vi "main_ctrl.vi"(8 "error in":errorcluster) -> (0 "error out":errorcluster caption="Error")   [LabVIEW 2013]
uses:
  <vilib>/Rock Robotics/WPI/DriverStation/WPI_DriverStationRobotMode2.ctl
  typedefs/fg_typedef.ctl
  typedefs/vision enable.ctl
  typedefs/vision data.ctl
  typedefs/subStates.ctl
  typedefs/singleUseSubstate.ctl
  <vilib>/Rock Robotics/WPI/Solenoid/WPI_SolenoidValue.ctl
  <vilib>/Rock Robotics/WPI/Compressor/WPI_CompressorGetSetRefNum.vi
  <vilib>/Rock Robotics/WPI/RobotDrive/WPI_RobotDriveGetSetRefNum.vi
  <vilib>/Rock Robotics/WPI/RobotDrive/WPI_RobotDriveArcadeDrive_Standard(NoSaturation).vi
  <vilib>/Rock Robotics/WPI/Solenoid/WPI_SolenoidSetEnum.vi
panel:
  out "Robot Mode":T1
  out "Vision SPI":u32
  out "Vision IPS":dbl
  out "Main IPS":dbl
  out "Main SPI":u32
  # "MAIN CONTROL"
  # "holds robot control code - dual parallel state machine"
  # "SPI: milliseconds per iteration\nIPS: iterations per second"
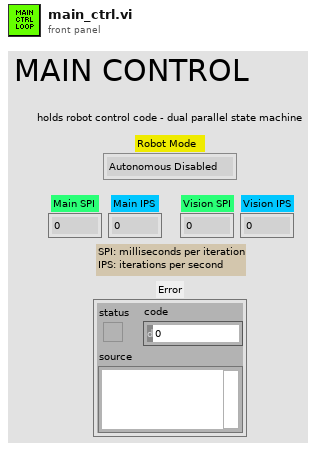
[diagram p1: front panel]
types:
  T1 = typedef "WPI_DriverStationRobotMode2.ctl" = enum16{"Autonomous Disabled", "Autonomous Enabled", "Teleop Disabled", "Teleop Enabled", "Timeout", "Finish", "Test Disabled", "Test Enabled"}
  T2 = typedef "fg_typedef.ctl" = enum16{"Get", "Set"}
  T3 = typedef "WPI_RobotDriveDevRef.ctl" = cluster{"DevStatus":errorcluster, "Motors[]":T4[], "Square Inputs":bool, "Max Output":dbl, "Isochronous":bool}
  T4 = typedef "WPI_MotorControlDeviceRef.ctl" = cluster{"DeviceStatus":errorcluster, "Type":enum16{"PWM", "CAN"}, "PWM":cluster{"Digital Module":T5, "PWM Channel":T6, "DeadBand":T7}, "CAN":cluster{"Device Number":u8, "Control Mode":T8, "Semaphore":T9, "Max Vout":dbl}, "Invert":bool, "TransformRef":T10, "InvTransformRef":T10}
  T5 = typedef "FPGA_TypedefDigitalModule.ctl" = enum16{"Digital Module 1", "Digital Module 2"}
  T6 = typedef "FPGA_DIOPWMChannel.ctl" = enum8{"PWM 1", "PWM 2", "PWM 3", "PWM 4", "PWM 5", "PWM 6", "PWM 7", "PWM 8", "PWM 9", "PWM 10", "Invalid"}
  T7 = typedef "WPI_PWMDeadband.ctl" = cluster{"Name":string, "maxPositivePwm":i32, "minPositivePwm":i32, "centerPwm":i32, "maxNegativePwm":i32, "minNegativePwm":i32, "angularRange":u16}
  T8 = typedef "WPI_CANJaguar_ControlMode.ctl" = enum8{"Percent VBus", "Current", "Speed", "Position", "Voltage"}
  T9 = typedef "Semaphore RefNum" = refnum<k1>
  T10 = typedef "WPI_PWMTransform_ConPane.ctl" = refnum<vi>
  T11 = typedef "WPI_SolenoidDevRef.ctl" = cluster{"DevStatus":errorcluster, "Solenoid Module":T12, "Forward Solenoid Channel":T13, "Reverse Solenoid Channel":T13}
  T12 = typedef "FPGA_TypedefSolenoidModule.ctl" = enum16{"Solenoid Module 1", "Solenoid Module 2"}
  T13 = typedef "WPI_SolenoidChannel.ctl" = enum8{"Solenoid 1", "Solenoid 2", "Solenoid 3", "Solenoid 4", "Solenoid 5", "Solenoid 6", "Solenoid 7", "Solenoid 8", "Invalid"}
  T14 = typedef "WPI_DigitalInputDevRef.ctl" = cluster{"DevStatus":errorcluster, "DIO Channel":T15, "Digital Module":T5}
  T15 = typedef "FPGA_DIOChannel.ctl" = enum8{"DIO 1", "DIO 2", "DIO 3", "DIO 4", "DIO 5", "DIO 6", "DIO 7", "DIO 8", "DIO 9", "DIO 10", "DIO 11", "DIO 12", "DIO 13", "DIO 14", "Invalid"}
  T16 = typedef "WPI_EncoderDevRef.ctl" = cluster{"DevStatus":errorcluster, "EncoderIndex":T17, "CounterIndex":T18, "DistancePerCount":dbl, "Decoding Type":T19}
  T17 = typedef "FPGA_EncoderIdx.ctl" = enum8{"Enc 0", "Enc 1", "Enc 2", "Enc 3", "Invalid"}
  T18 = typedef "FPGA_CounterCtrSystemIndex.ctl" = enum8{"Ctr 0", "Ctr 1", "Ctr 2", "Ctr 3", "Ctr 4", "Ctr 5", "Ctr 6", "Ctr 7", "Invalid"}
  T19 = typedef "WPI_EncoderType.ctl" = enum16{"1x", "2x", "4x"}
  T20 = typedef "vision data.ctl" = cluster{"x":dbl, "y":dbl, "area":dbl, "width":dbl, "height":dbl, "Hot Goal Present?":bool, "distance":dbl}
  T21 = typedef "vision enable.ctl" = enum16{"Enable", "Disable", "Stop"}
  T22 = typedef "WPI_CameraDevRef.ctl" = cluster{"Camera Address":string, "CameraStatus":errorcluster, "Acquire Image Notifier":refnum<notifier>}
  T23 = typedef "IMAQ Image.ctl" = refnum<image>
  T24 = cluster{"Vision mSPI":u32, "Main mSPI":u32, "Dash mSPI":u32}
  T25 = typedef "WPI_CompressorDevRef.ctl" = cluster{"DevStatus":errorcluster, "DigitalInputDevRef":T14, "RelayDevRef":T26}
  T26 = typedef "WPI_RelayDevRef.ctl" = cluster{"DevStatus":errorcluster, "Relay Channel":T27, "Digital Module":T5, "Relay Direction":T28}
  T27 = typedef "FPGA_DIORelayChannel.ctl" = enum8{"Relay 1", "Relay 2", "Relay 3", "Relay 4", "Relay 5", "Relay 6", "Relay 7", "Relay 8", "Invalid"}
  T28 = typedef "WPI_RelayDirection.ctl" = enum16{"Both directions", "Forward only", "Reverse only"}
  T29 = typedef "WPI_SolenoidValue.ctl" = enum16{"Off", "On", "Forward", "Reverse"}
  T30 = typedef "singleUseSubstate.ctl" = enum16{"null", "wait", "shift high", "shift low", "extend shooter", "retract shooter", "latch", "unlatch"}
  T31 = typedef "WPI_DriverStationDerivedRobotMode.ctl" = enum16{"Init", "Execute", "Stop"}
  T32 = typedef "subStates.ctl" = enum16{"null", "wait", "driver control", "auto", "manual override", "hold position", "rotate", "pickup", "pass", "load", "goto shoot", "shoot high goal", "shoot low goal", "cancel arm", "cancel shooter", "end"}
  T33 = typedef "Loop 2 Datatype.ctl" = cluster{"State":T32, "Waiting Loop":i32, "State to Wait For":i32, "Loop ID":i32, "Exit Value":i32, "Joystick Y":dbl, "Joystick Z":dbl}
  T34 = typedef "Loop 1 Datatype.ctl" = cluster{"State":T32, "Waiting Loop":i32, "State to Wait For":i32, "Loop ID":i32, "Exit Value":i32}
  T35 = typedef "Loop 3 Datatype.ctl" = cluster{"State":T32, "Waiting Loop":i32, "State to Wait For":i32, "Loop ID":i32, "Exit Value":i32, "Joystick Y":dbl, "Tune Setpoint":cluster{"Increment":bool, "Decrement":bool}}
  T36 = typedef "Loop 0 Datatype.ctl" = cluster{"State":T32, "Waiting Loop":i32, "State to Wait For":i32, "Loop ID":i32, "Exit Value":i32, "X Axis":dbl, "Y Axis":dbl, "Z Axis":dbl}
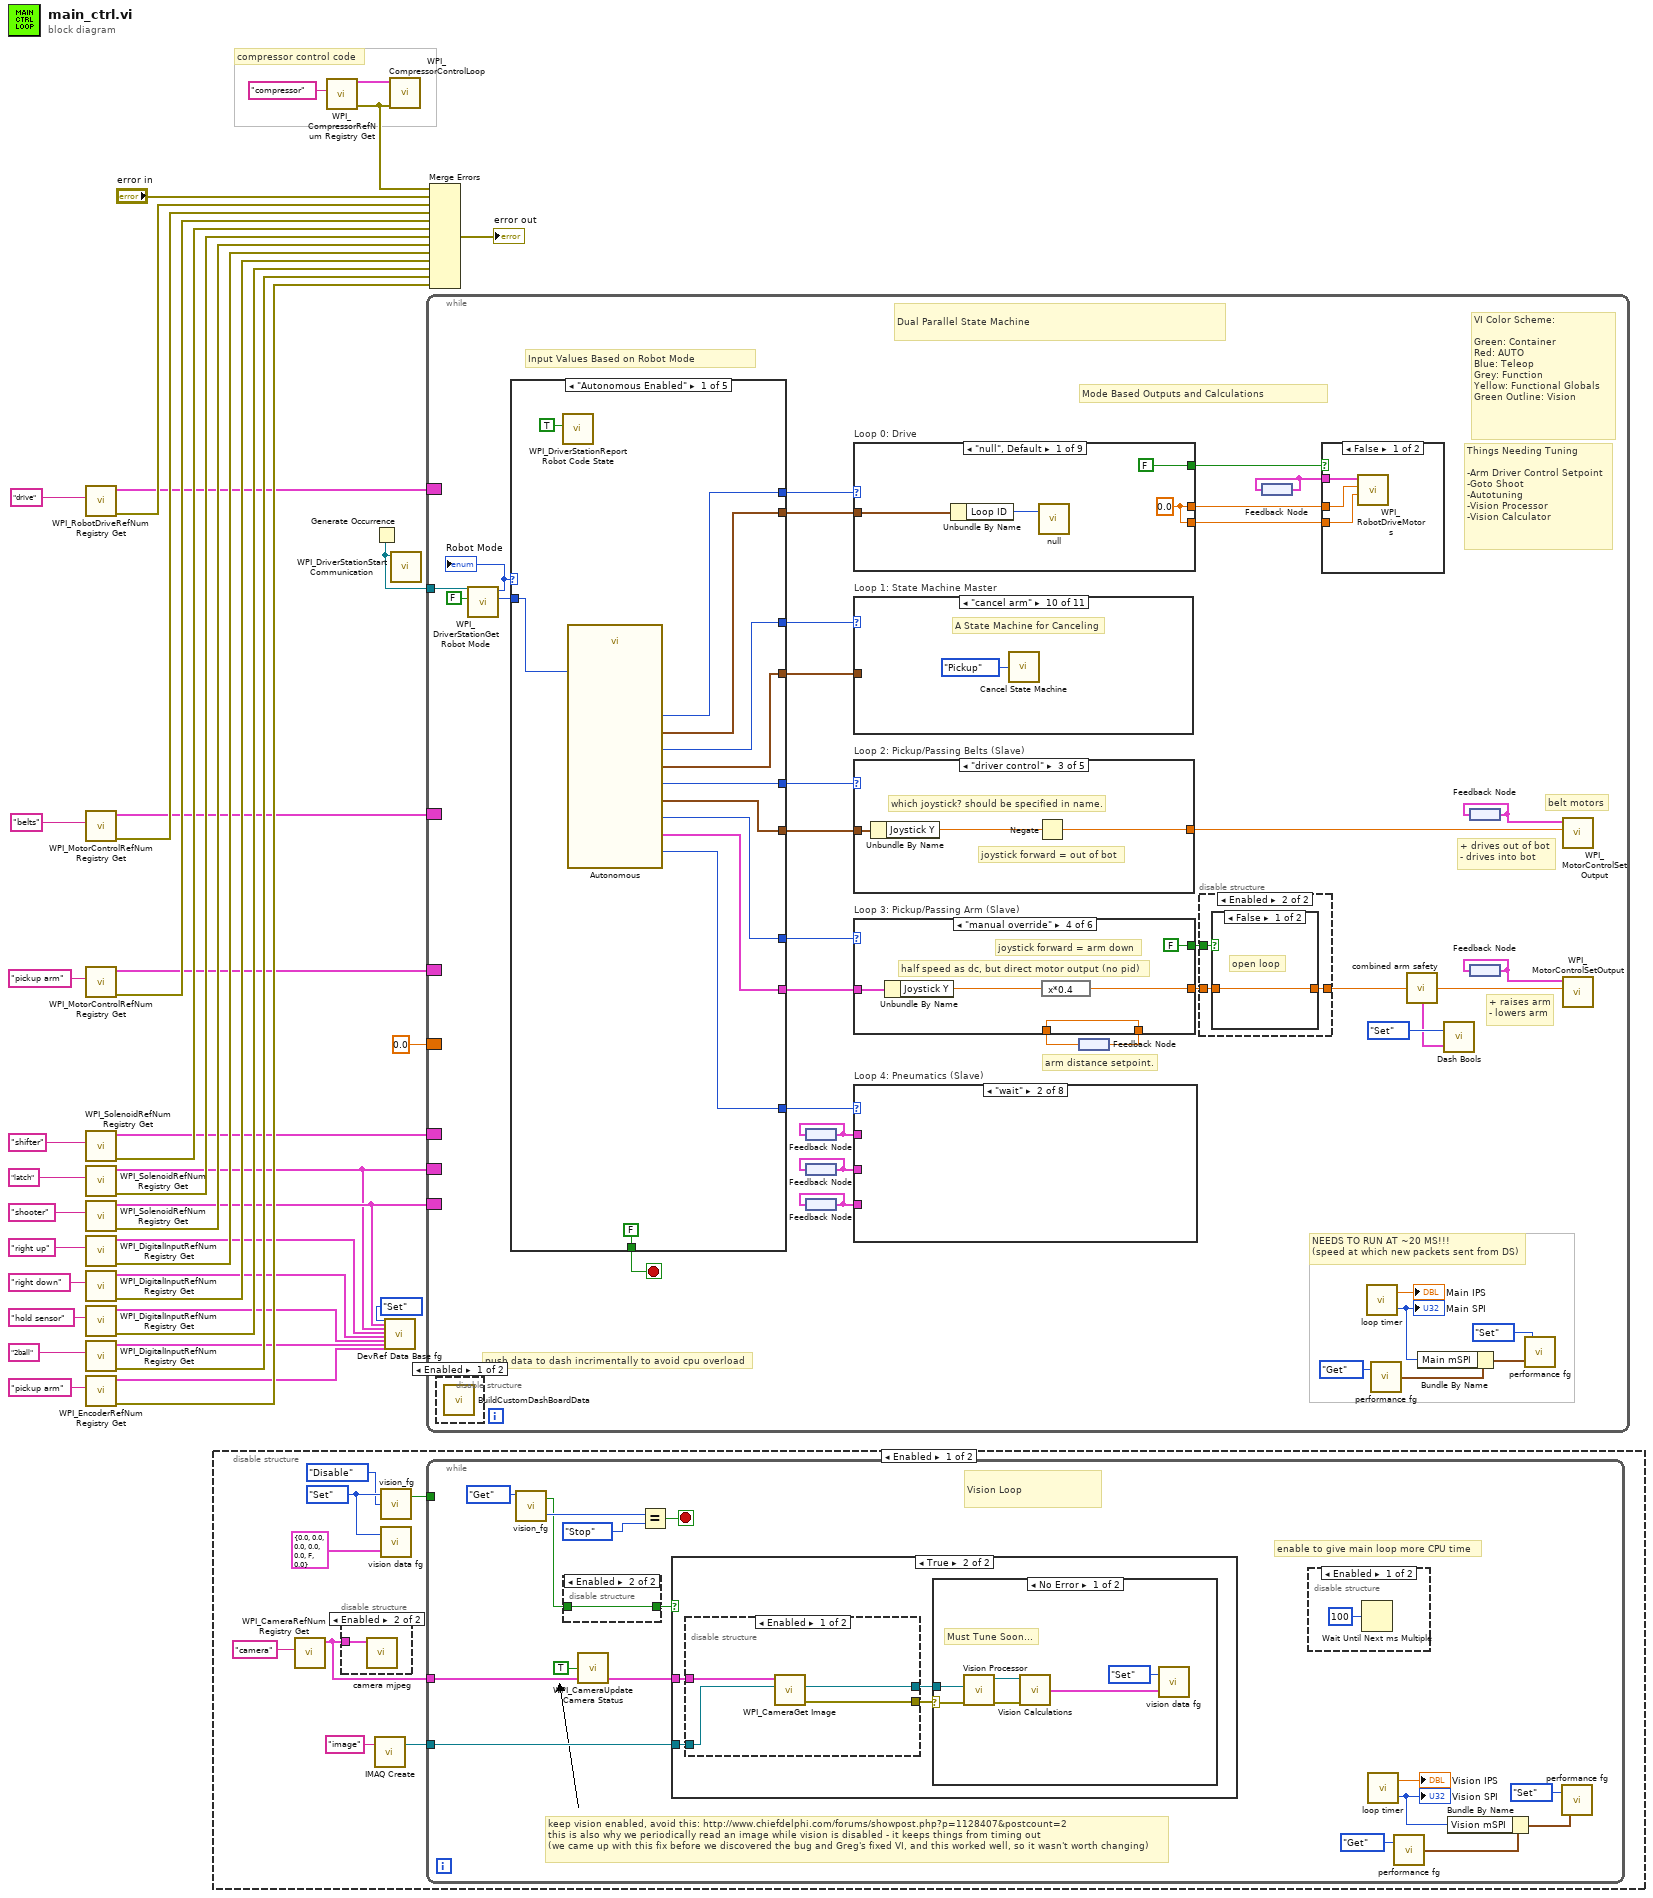
[diagram p0: block diagram]
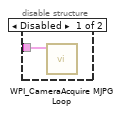
[diagram p2: hidden frame]
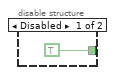
[diagram p3: hidden frame]
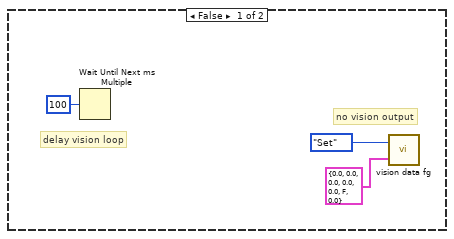
[diagram p5: hidden frame]
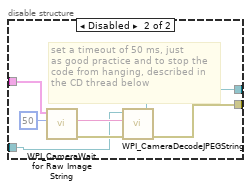
[diagram p7: hidden frame]
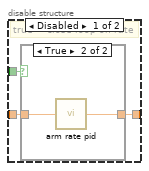
[diagram p9: hidden frame]
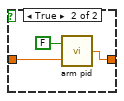
[diagram p11: hidden frame]
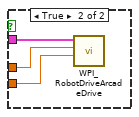
[diagram p13: hidden frame]
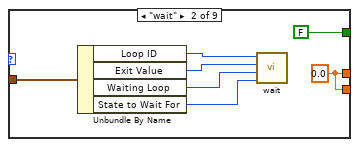
[diagram p14: hidden frame]
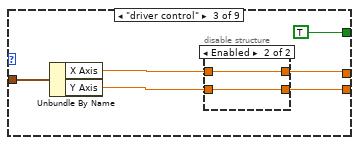
[diagram p15: hidden frame]
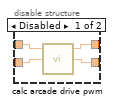
[diagram p16: hidden frame]
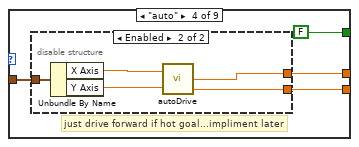
[diagram p17: hidden frame]
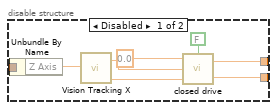
[diagram p18: hidden frame]
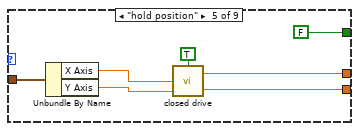
[diagram p19: hidden frame]
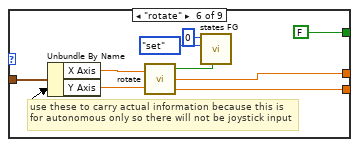
[diagram p20: hidden frame]
diagram:
  # "compressor control code"
  n1 = call <vilib>:"WPI_RobotDriveRefNum Registry Get.vi"("refnum name"="drive") -> ("error out"=w39:errorcluster, "RobotDriveDevRef"=w27:T3)  [unwired: 9 in]
  n2 = call <vilib>:"WPI_MotorControlRefNum Registry Get.vi"("refnum name"="belts") -> ("error out"=w38:errorcluster, "MotorControlDevRef"=w1:T4)  [unwired: 9 in]
  n3 = call <vilib>:"WPI_MotorControlRefNum Registry Get.vi"("refnum name"="pickup arm") -> ("error out"=w37:errorcluster, "MotorControlDevRef"=w18:T4)  [unwired: 9 in]
  n4 = call <vilib>:"WPI_SolenoidRefNum Registry Get.vi"("refnum name"="shifter") -> ("error out"=w36:errorcluster, "SolenoidDevRef"=w25:T11)  [unwired: 9 in]
  n5 = call <vilib>:"WPI_SolenoidRefNum Registry Get.vi"("refnum name"="latch") -> ("error out"=w35:errorcluster, "SolenoidDevRef"=w13:T11)  [unwired: 9 in]
  n6 = call <vilib>:"WPI_SolenoidRefNum Registry Get.vi"("refnum name"="shooter") -> ("error out"=w34:errorcluster, "SolenoidDevRef"=w14:T11)  [unwired: 9 in]
  n7 = call <vilib>:"WPI_DigitalInputRefNum Registry Get.vi"("refnum name"="right up") -> ("error out"=w33:errorcluster, "DigitalInputDevRef"=w12:T14)  [unwired: 9 in]
  n8 = call <vilib>:"WPI_DigitalInputRefNum Registry Get.vi"("refnum name"="right down") -> ("error out"=w32:errorcluster, "DigitalInputDevRef"=w11:T14)  [unwired: 9 in]
  n9 = call <vilib>:"WPI_DigitalInputRefNum Registry Get.vi"("refnum name"="hold sensor") -> ("error out"=w31:errorcluster, "DigitalInputDevRef"=w8:T14)  [unwired: 9 in]
  n10 = call <vilib>:"WPI_DigitalInputRefNum Registry Get.vi"("refnum name"="2ball") -> ("error out"=w40:errorcluster, "DigitalInputDevRef"=w3:T14)  [unwired: 9 in]
  n11 = call <vilib>:"WPI_EncoderRefNum Registry Get.vi"("refnum name"="pickup arm") -> ("error out"=w41:errorcluster, "EncoderDevRef"=w2:T16)  [unwired: 9 in]
  n12 = disable-structure shown="Enabled" {
    frame Enabled {
      w47 = fg_typedef."Set" ("Enum")
      n13 = call <vilib>:"WPI_CameraRefNum Registry Get.vi"("refnum name"="camera") -> ("CameraDevRef"=w44:T22)  [unwired: 9 in, 1 out]
      n14 = disable-structure shown="Enabled" {
        disable-tunnel: w44 -> [w50 w51]
        frame Disabled {
          n15 = call <vilib>:"WPI_CameraAcquire MJPG Loop.vi"("CameraDevRef"=w50) -> ()  [unwired: 11 in]
        }
        frame Enabled {
          n16 = call "camera mjpeg.vi"("CameraDevRef"=w51) -> ()  [unwired: 11 in]
        }
      }
      n17 = call "IMAQ Create"("Image Name"="image") -> ("New Image"=w49:T23)  [unwired: 4 in, 1 out]
      n18 = call "vision_fg.vi"("Action"=vision_enable."Disable", "Menu"=w47) -> ("Enabled?"=w48:bool)  [unwired: 1 in, 1 out]
      n19 = call "vision data fg.vi"("Input"=T20 {"x"=0.0, "y"=0.0, "area"=0.0, "width"=0.0, "height"=0.0, "Hot Goal Present?"=FALSE, "distance"=0.0} ("Cluster"), "Menu"=w47) -> ()  [unwired: 1 out]
      n20 = while {
        tunnel: w49 -> [w66]
        tunnel: w44 -> [w65]
        tunnel: w48 -> [_]
        stop <- w67 stop-if-true
        # "keep vision enabled, avoid this: http://www.chiefdelphi.com/forums/showpost.php?p=1128407&postcount=2\nthis is also why we periodically read an image while vision is disabled - it keeps things from timing out\n(we came up with this fix before we discovered the bug and Greg's fixed VI, and this worked well, so it wasn't worth changing)"
        # "enable to give main loop more CPU time"
        # "Vision Loop"
        n21 = call "vision_fg.vi"("Menu"=fg_typedef."Get" ("Enum")) -> ("State Out"=w61:T21, "Enabled?"=w52:bool)  [unwired: 2 in]
        n22 = disable-structure shown="Enabled" {
          disable-tunnel: [TRUE w69] -> w53
          disable-tunnel: w52 -> [_ w69]
          frame Disabled {
          }
          frame Enabled {
          }
        }
        n23 = call <vilib>:"WPI_CameraUpdate Camera Status.vi"("CameraDevRef In"=w65, "Enable Vision"=TRUE) -> ("CameraDevRef Out"=w64:T22)  [unwired: 3 in]
        n24 = Equal?(x=w61, y=vision_enable."Stop") -> (x = y?=w67:bool)
        n25 = case shown="True" w53 {
          tunnel: w66 -> [_ w77]
          tunnel: w64 -> [_ w76]
          frame False {
            # "no vision output"
            # "delay vision loop"
            n26 = Wait Until Next ms Multiple(millisecond multiple=u32 100) -> ()  [unwired: 1 out]
            n27 = call "vision data fg.vi"("Input"=T20 {"x"=0.0, "y"=0.0, "area"=0.0, "width"=0.0, "height"=0.0, "Hot Goal Present?"=FALSE, "distance"=0.0} ("Cluster"), "Menu"=fg_typedef."Set" ("Enum")) -> ()  [unwired: 1 out]
          }
          frame True {
            n28 = disable-structure shown="Enabled" {
              disable-tunnel: w77 -> [w86 w90]
              disable-tunnel: w76 -> [w87 w92]
              disable-tunnel: [w85 w89] -> w75
              disable-tunnel: [w84 w88] -> w74
              frame Enabled {
                n29 = call <vilib>:"WPI_CameraGet Image.vi"("Image"=w86, "CameraDevRef"=w87) -> ("error out"=w84:errorcluster, "Image Out"=w85:T23)  [unwired: 7 in, 1 out]
              }
              frame Disabled {
                # "set a timeout of 50 ms, just\nas good practice and to stop the \ncode from hanging, described in \nthe CD thread below"
                n30 = call <vilib>:"WPI_CameraWait for Raw Image String.vi"("Timeout in ms (-1)"=50, "CameraDevRef"=w92) -> ("error out"=w94:errorcluster, "String"=w93:string)  [unwired: 3 in, 5 out]
                n31 = call <vilib>:"WPI_CameraDecodeJPEGString.vi"("error in"=w94, "Compressed Image"=w93, "Image In"=w90) -> ("error out"=w88:errorcluster, "Image Out"=w89:T23)  [unwired: 3 out]
              }
            }
            n32 = case shown="No Error" w74 {
              selector: w74 -> [w82 _]
              tunnel: w75 -> [w81 _]
              frame No Error {
                # "Must Tune Soon..."
                n33 = call "Vision Processor.vi"("error in"=w82, "Image In"=w81) -> ("error out"=w79:errorcluster, "Image Out"=w80:T23)  [unwired: 5 in]
                n34 = call "Vision Calculations.vi"("Image In"=w80, "error in"=w79) -> ("Vision Data"=w78:T20)  [unwired: 3 in]
                n35 = call "vision data fg.vi"("Input"=w78, "Menu"=fg_typedef."Set" ("Enum")) -> ()  [unwired: 1 out]
              }
              frame Error {
              }
            }
          }
        }
        n36 = disable-structure shown="Enabled" {
          frame Enabled {
            n37 = Wait Until Next ms Multiple(millisecond multiple=u32 100) -> ()  [unwired: 1 out]
          }
          frame Disabled {
          }
        }
        n38 = call "loop timer.vi"() -> ("IPS"=→"Vision IPS":dbl, "SPI"=w59:u32)  [unwired: 1 in]
        "Vision SPI" <- w59
        n39 = call "performance fg.vi"("Menu"=fg_typedef."Get") -> ("Output"=w57:T24)  [unwired: 1 in]
        n40 = Bundle By Name(cluster=w57, "Vision mSPI"=w59) -> (w56:T24)
        n41 = call "performance fg.vi"("Input"=w56, "Menu"=fg_typedef."Set") -> ()  [unwired: 1 out]
      }
    }
    frame Disabled {
      # "no vision at suffield"
    }
  }
  n42 = call <vilib>:"WPI_CompressorRefNum Registry Get.vi"("refnum name"="compressor") -> ("error out"=w7:errorcluster, "CompressorDevRef"=w26:T25)  [unwired: 9 in]
  n43 = Generate Occurrence() -> (w23:refnum<k4>)
  n44 = call "DevRef Data Base fg.vi"("Menu"=fg_typedef."Set", "Shooter Solenoid DevRef"=w14, "Latch Solenoid DevRef"=w13, "Right Up DevRef"=w12, "Right Down DevRef"=w11, "Hold Sensor DevRef"=w8, "2 Ball DevRef"=w3, "Arm Encoder DevRef"=w2) -> ()  [unwired: 17 in, 3 out]
  n45 = call <vilib>:"WPI_CompressorControlLoop.vi"("error in (no error)"=w7, "CompressorDevRef"=w26) -> ()  [unwired: 10 in]
  n46 = call <vilib>:"WPI_DriverStationStart Communication.vi"("occurrence"=w23) -> ()  [unwired: 11 in]
  n47 = while {
    tunnel: w23 -> [w110]
    border: w27 -> [_]
    border: w25 -> [_]
    border: w14 -> [_]
    border: w13 -> [_]
    border: w1 -> [_]
    border: w18 -> [_]
    border: 0.0 ("setpoint") -> [_]
    stop <- w129 stop-if-true
    # "arm distance setpoint."
    # "push data to dash incrimentally to avoid cpu overload"
    # "Things Needing Tuning\n\n-Arm Driver Control Setpoint\n-Goto Shoot\n-Autotuning\n-Vision Processor\n-Vision Calculator"
    # "+ raises arm\n- lowers arm"
    # "+ drives out of bot\n- drives into bot"
    # "belt motors"
    # "VI Color Scheme:\n\nGreen: Container\nRed: AUTO\nBlue: Teleop\nGrey: Function\nYellow: Functional Globals\nGreen Outline: Vision"
    # "Input Values Based on Robot Mode"
    # "Mode Based Outputs and Calculations"
    # "NEEDS TO RUN AT ~20 MS!!!\n(speed at which new packets sent from DS)"
    # "Dual Parallel State Machine"
    n48 = disable-structure shown="Enabled" {
      frame Enabled {
        n49 = call "BuildCustomDashBoardData.vi"() -> ()  [unwired: 12 in]
      }
      frame Disabled {
      }
    }
    n50 = call <vilib>:"WPI_DriverStationGet Robot Mode.vi"("Finish"=FALSE, "DS Occurrence"=w110) -> ("Call Context"=w109:T31, "Robot Mode"=w108:T1)  [unwired: 8 out]
    "Robot Mode" <- w108
    n51 = case shown="\"Autonomous Enabled\"" w108 {
      tunnel: [w309 w324 w327 w333 w339] -> w112
      tunnel: w109 -> [w302 w320 _ _ _]
      tunnel: [w307 w323 w327 w333 w339] -> w131
      tunnel: [w303 w321 singleUseSubstate."null" ("SubState 5") singleUseSubstate."null" ("SubState 5") singleUseSubstate."null" ("SubState 5")] -> w130
      tunnel: [FALSE FALSE FALSE FALSE TRUE] -> w129
      tunnel: [w311 w319 w327 w333 w339] -> w122
      tunnel: [w310 w318 _ _ _] -> w123
      tunnel: [w308 w317 _ _ _] -> w121
      tunnel: [w306 w316 _ _ _] -> w120
      tunnel: [w304 w315 _ _ _] -> w118
      tunnel: [w305 w314 w327 w333 w339] -> w117
      frame "Autonomous Enabled" {
        n52 = call <vilib>:"WPI_DriverStationReport Robot Code State.vi"("Autonomous"=TRUE) -> ()  [unwired: 10 in, 1 out]
        n53 = call "Autonomous.vi"("Call Context"=w302) -> ("SubState 2"=w307:T32, "Loop 2 Data"=w306:T33, "SubState 1"=w309:T32, "Loop 1 Data"=w308:T34, "Loop 3 Data"=w304:T35, "SubState 0"=w311:T32, "SubState 3"=w305:T32, "Loop 0 Data"=w310:T36, "SubState 4"=w303:T30)  [unwired: 2 in]
      }
      frame "Teleop Enabled" {
        n54 = call <vilib>:"WPI_DriverStationReport Robot Code State.vi"("TeleOp"=TRUE) -> ()  [unwired: 10 in, 1 out]
        n55 = call "Teleop.vi"("Call Context"=w320) -> ("SubState 3"=w314:T32, "SubState 4"=w321:T30, "Loop 3 Data"=w315:T35, "SubState 0"=w319:T32, "Loop 1 Data"=w317:T34, "Loop 0 Data"=w318:T36, "SubState 1"=w324:T32, "Loop 2 Data"=w316:T33, "SubState 2"=w323:T32)  [unwired: 10 in]
      }
      frame "Autonomous Disabled", "Teleop Disabled", "Timeout" {
        w327 = subStates."null" ("SubState 0")
        # "set all loops to null"
        # "make sure to disable vision\nwe don't need it here"
        # "robot disabled, timeout"
        n56 = call <vilib>:"WPI_DriverStationReport Robot Code State.vi"("Disabled"=TRUE) -> ()  [unwired: 10 in, 1 out]
        n57 = call "vision_fg.vi"("Action"=vision_enable."Disable", "Menu"=fg_typedef."Set") -> ()  [unwired: 1 in, 2 out]
      }
      frame "Test Disabled", "Test Enabled" {
        w333 = subStates."null" ("SubState 0")
        # "set all loops to null"
        # "make sure to disable vision\nwe don't need it here"
        # "test, unused"
        n58 = call <vilib>:"WPI_DriverStationReport Robot Code State.vi"("Test"=TRUE) -> ()  [unwired: 10 in, 1 out]
        n59 = call "vision_fg.vi"("Action"=vision_enable."Disable", "Menu"=fg_typedef."Set") -> ()  [unwired: 1 in, 2 out]
      }
      frame "Finish" {
        w339 = subStates."end"  # Stop All Loops
        # "stop the while loop"
        # "stop DS comms"
        # "stop vision loop"
        n60 = call <vilib>:"WPI_DriverStationStop Communication.vi"("StopCommunication"=TRUE) -> ()  [unwired: 10 in, 1 out]
        n61 = call "vision_fg.vi"("Action"=vision_enable."Stop", "Menu"=fg_typedef."Set") -> ()  [unwired: 1 in, 2 out]
      }
    }
    n62 = feedback #1() -> (w119:T11)
    n63 = feedback-in #1(w119) -> ()
    n64 = feedback #2() -> (w96:T11)
    n65 = feedback-in #2(w96) -> ()
    n66 = feedback #3() -> (w95:T11)
    n67 = feedback-in #3(w95) -> ()
    n68 = case "Loop 0: Drive" shown="\"null\", Default" w122 {
      tunnel: w123 -> [w154 w158 w168 w175 w197 w204 _ _ w222]
      tunnel: [w152 w156 w166 w177 w194 w206 w209 w216 w218] -> w115
      tunnel: [w152 w156 w165 w176 w193 w205 w208 w216 w217] -> w114
      tunnel: [FALSE FALSE TRUE FALSE FALSE FALSE FALSE FALSE FALSE] -> w116
      frame "null", Default {
        w152 = 0.0 ("X Axis")
        n69 = Unbundle By Name(w154) -> ("Loop ID"=w155:i32)
        n70 = call "null.vi"("This Loop ID"=w155) -> ()  [unwired: 2 in]
      }
      frame "wait" {
        w156 = 0.0 ("X Axis")
        n71 = Unbundle By Name(w158) -> ("Loop ID"=w162:i32, "Exit Value"=w161:i32, "Waiting Loop"=w160:i32, "State to Wait For"=w159:i32)
        n72 = call "wait.vi"("State to wait for"=w159, "Waiting Loop ID"=w160, "time (ms)"=w161, "Current Loop ID"=w162) -> ()  [unwired: 1 out]
      }
      frame "driver control" {
        n73 = Unbundle By Name(w168) -> ("X Axis"=w163:dbl, "Y Axis"=w164:dbl)
        n74 = disable-structure shown="Enabled" {
          disable-tunnel: w163 -> [w172 w174]
          disable-tunnel: w164 -> [w171 w173]
          disable-tunnel: [w170 w174] -> w166
          disable-tunnel: [w169 w173] -> w165
          frame Disabled {
            n75 = call "calc arcade drive pwm.vi"("Y axis value"=w171, "X axis value"=w172) -> ("Right Speed"=w169:dbl, "Left Speed"=w170:dbl)  [unwired: 1 in, 1 out]
          }
          frame Enabled {
          }
        }
      }
      frame "auto" {
        # "just drive forward if hot goal...impliment later"
        n76 = disable-structure shown="Enabled" {
          disable-tunnel: [w186 w191] -> w177
          disable-tunnel: [w185 w190] -> w176
          disable-tunnel: w175 -> [w181 w189]
          frame Disabled {
            n77 = Unbundle By Name(w181) -> ("Z Axis"=w179:dbl)
            n78 = call "Vision Tracking X.vi"("Tweak"=w179) -> ("right speed"=w180:dbl, "left speed"=w183:dbl)
            n79 = call "closed drive.vi"("Acrade Drive?"=FALSE, "Y axis value (Left)"=w183, "X axis value (Right)"=w180, "Threshold (.4)"=0.0 ("Threshold")) -> ("right"=w185:dbl, "left"=w186:dbl)
          }
          frame Enabled {
            n80 = Unbundle By Name(w189) -> ("X Axis"=w188:dbl, "Y Axis"=w187:dbl)
            n81 = call "autoDrive.vi"("Distance to Travel"=w188, "Rate"=w187) -> ("left speed"=w191:dbl, "right speed"=w190:dbl)  [unwired: 1 out]
          }
        }
      }
      frame "hold position" {
        n82 = Unbundle By Name(w197) -> ("X Axis"=w196:dbl, "Y Axis"=w195:dbl)
        n83 = call "closed drive.vi"("Acrade Drive?"=TRUE, "Y axis value (Left)"=w195, "X axis value (Right)"=w196) -> ("right"=w193:dbl, "left"=w194:dbl)  [unwired: 1 in]
      }
      frame "rotate" {
        # "use these to carry actual information because this is\nfor autonomous only so there will not be joystick input"
        n84 = Unbundle By Name(w204) -> ("X Axis"=w203:dbl, "Y Axis"=w202:dbl)
        n85 = call "rotate.vi"("Angle"=w203, "Rate"=w202) -> ("finished?"=w199:bool, "left speed"=w206:dbl, "right speed"=w205:dbl)
        n86 = call "states FG.vi"("exit in"=w199, "menu (get)"=enum16{"set", "get"}."set", "Loop ID"=0) -> ()  [unwired: 5 in, 4 out]
      }
      frame "goto shoot" {
        n87 = disable-structure shown="Disabled" {
          disable-tunnel: [w212 _] -> w209
          disable-tunnel: [w211 _] -> w208
          frame Disabled {
            # "consider implimenting closed hold with drive"
            n88 = call "vision data fg.vi"("Menu"=fg_typedef."Get") -> ("Output"=w213:T20)  [unwired: 1 in]
            n89 = call "goto location.vi"("Image Data"=w213) -> ("left speed"=w212:dbl, "right speed"=w211:dbl)
          }
          frame Enabled {
            # "not going to do this"
          }
        }
      }
      frame "end" {
        w216 = 0.0 ("X Axis")
      }
      frame "manual override" {
        n90 = Unbundle By Name(w222) -> ("X Axis"=w221:dbl, "Y Axis"=w220:dbl)
        n91 = expression code="x/2"(w221) -> (w218:dbl)
        n92 = expression code="x/2"(w220) -> (w217:dbl)
      }
    }
    n93 = case "Loop 1: State Machine Master" shown="\"cancel arm\"" w112 {
      tunnel: w121 -> [w289 w291 _ _ _ _ _ _ _ _ _]
      frame "null", Default {
        n94 = Unbundle By Name(w289) -> ("Loop ID"=w290:i32)
        n95 = call "null.vi"("This Loop ID"=w290) -> ()  [unwired: 2 in]
      }
      frame "wait" {
        n96 = Unbundle By Name(w291) -> ("Loop ID"=w295:i32, "Exit Value"=w294:i32, "Waiting Loop"=w293:i32, "State to Wait For"=w292:i32)
        n97 = call "wait.vi"("State to wait for"=w292, "Waiting Loop ID"=w293, "time (ms)"=w294, "Current Loop ID"=w295) -> ()  [unwired: 1 out]
      }
      frame "auto" {
        # "A State Machine for Auto"
        n98 = call "Auto State Machine.vi"() -> ()  [unwired: 12 in]
      }
      frame "manual override" {
        # "manual shoot"
        n99 = call "single use states FG.vi"("exit in"=TRUE, "substate"=singleUseSubstate."unlatch", "menu (get)"=enum16{"set", "get"}."set") -> ()  [unwired: 5 in, 4 out]
      }
      frame "pickup" {
        # "A State Machine for Pickup"
        n100 = call "Pickup State Machine.vi"() -> ()  [unwired: 12 in]
      }
      frame "pass" {
        # "A State Machine for Passing"
        n101 = call "Pass State Machine.vi"() -> ()  [unwired: 12 in]
      }
      frame "load" {
        # "ball can now (after this) be high or low goal shot"
        # "A State Machine for Loading"
        n102 = call "Load State Machine.vi"() -> ()  [unwired: 12 in]
      }
      frame "shoot high goal" {
        # "A State Machine for High Goal Shooting"
        n103 = call "Shoot High Goal State Machine.vi"() -> ()  [unwired: 12 in]
      }
      frame "shoot low goal" {
        # "A State Machine for Low Goal Shooting"
        n104 = call "Shoot Low Goal State Machine.vi"() -> ()  [unwired: 12 in]
      }
      frame "cancel arm" {
        # "A State Machine for Canceling"
        n105 = call "Cancel State Machine.vi"("What to Cancel"=enum16{"Pickup", "Load"}."Pickup") -> ()
      }
      frame "cancel shooter" {
        # "A State Machine for Canceling"
        n106 = call "Cancel State Machine.vi"("What to Cancel"=enum16{"Pickup", "Load"}."Load") -> ()
      }
    }
    n107 = case "Loop 2: Pickup/Passing Belts (Slave)" shown="\"driver control\"" w131 {
      tunnel: w120 -> [w269 w271 w278 w281 w288]
      tunnel: [0.0 ("output") 0.0 ("output") w276 w279 w285] -> w99
      frame "null", Default {
        n108 = Unbundle By Name(w269) -> ("Loop ID"=w268:i32)
        n109 = call "null.vi"("This Loop ID"=w268) -> ()  [unwired: 2 in]
      }
      frame "wait" {
        n110 = Unbundle By Name(w271) -> ("Loop ID"=w275:i32, "Exit Value"=w274:i32, "Waiting Loop"=w273:i32, "State to Wait For"=w272:i32)
        n111 = call "wait.vi"("State to wait for"=w272, "Waiting Loop ID"=w273, "time (ms)"=w274, "Current Loop ID"=w275) -> ()  [unwired: 1 out]
      }
      frame "driver control" {
        # "which joystick? should be specified in name."
        # "joystick forward = out of bot"
        n112 = Unbundle By Name(w278) -> ("Joystick Y"=w277:dbl)
        n113 = Negate(x=w277) -> (-x=w276:dbl)
      }
      frame "manual override" {
        # "essentially driver control, but 1/2 speed?"
        # "joystick forward = out of bot"
        n114 = Unbundle By Name(w281) -> ("Joystick Y"=w280:dbl)
        n115 = expression code="-x/2"(w280) -> (w279:dbl)
      }
      frame "auto" {
        # "get speed to go as set by master and tune"
        n116 = Unbundle By Name(w288) -> ("Joystick Z"=w286:dbl)
        n117 = call "Joystick tuner.vi"("Joystick Z"=w286, "Loop ID"=2) -> ("Output"=w284:dbl)  [unwired: 7 in]
        n118 = call "Belt Speed FG.vi"("Menu"=fg_typedef."Get") -> ("Speed Out"=w283:dbl)  [unwired: 1 in]
        n119 = Multiply(x=w284, y=w283) -> (x*y=w285:dbl)
      }
    }
    n120 = case "Loop 4: Pneumatics (Slave)" shown="\"wait\"" w130 {
      tunnel: w119 -> [_ _ w256 w257 _ _ _ _]
      tunnel: w96 -> [_ _ _ _ w259 w261 _ _]
      tunnel: w95 -> [_ _ _ _ _ _ w263 w265]
      frame "null", Default {
      }
      frame "wait" {
      }
      frame "shift high" {
        n121 = call-poly <vilib>:"WPI_SolenoidSet.vi"("Value"=WPI_SolenoidValue."Forward", "SolenoidDevRef"=w256) -> ()  [unwired: 8 in, 2 out]
      }
      frame "shift low" {
        n122 = call-poly <vilib>:"WPI_SolenoidSet.vi"("Value"=WPI_SolenoidValue."Reverse", "SolenoidDevRef"=w257) -> ()  [unwired: 8 in, 2 out]
      }
      frame "extend shooter" {
        n123 = call-poly <vilib>:"WPI_SolenoidSet.vi"("Value"=WPI_SolenoidValue."Forward", "SolenoidDevRef"=w259) -> ()  [unwired: 8 in, 2 out]
      }
      frame "retract shooter" {
        n124 = call-poly <vilib>:"WPI_SolenoidSet.vi"("Value"=WPI_SolenoidValue."Reverse", "SolenoidDevRef"=w261) -> ()  [unwired: 8 in, 2 out]
      }
      frame "latch" {
        # "When the latch piston\nis reversed, the latch\nis closed. When the\nlatch piston is\nextended, the latch is\nopen."
        n125 = call-poly <vilib>:"WPI_SolenoidSet.vi"("Value"=WPI_SolenoidValue."Reverse", "SolenoidDevRef"=w263) -> ()  [unwired: 8 in, 2 out]
      }
      frame "unlatch" {
        # "When the latch piston\nis reversed, the latch\nis closed. When the\nlatch piston is\nextended, the latch is\nopen."
        n126 = call-poly <vilib>:"WPI_SolenoidSet.vi"("Value"=WPI_SolenoidValue."Forward", "SolenoidDevRef"=w265) -> ()  [unwired: 8 in, 2 out]
      }
    }
    n127 = feedback #4() -> (w100:dbl)
    n128 = case "Loop 3: Pickup/Passing Arm (Slave)" shown="\"manual override\"" w117 {
      tunnel: w118 -> [w227 w231 w239 w245 w252 _]
      tunnel: [FALSE FALSE TRUE FALSE TRUE TRUE] -> w105
      tunnel: [0.0 ("output") 0.0 ("output") w237 w243 w246 w253] -> w104
      tunnel: [w223 w228 w238 w241 w246 w253] -> w101
      tunnel: w100 -> [w223 w228 w238 w241 _ w253]
      frame "null", Default {
        n129 = Unbundle By Name(w227) -> ("Loop ID"=w226:i32)
        n130 = call "null.vi"("This Loop ID"=w226) -> ()  [unwired: 2 in]
      }
      frame "wait" {
        n131 = Unbundle By Name(w231) -> ("Loop ID"=w235:i32, "Exit Value"=w234:i32, "Waiting Loop"=w233:i32, "State to Wait For"=w232:i32)
        n132 = call "wait.vi"("State to wait for"=w232, "Waiting Loop ID"=w233, "time (ms)"=w234, "Current Loop ID"=w235) -> ()  [unwired: 1 out]
      }
      frame "driver control" {
        # "joystick forward = arm down"
        n133 = Unbundle By Name(w239) -> ("Joystick Y"=w236:dbl)
        n134 = call "arm driver control.vi"("Joystick Y"=w236) -> ("Setpoint"=w237:dbl)
      }
      frame "manual override" {
        # "half speed as dc, but direct motor output (no pid)"
        # "joystick forward = arm down"
        n135 = Unbundle By Name(w245) -> ("Joystick Y"=w244:dbl)
        n136 = expression code="x*0.4"(w244) -> (w243:dbl)
      }
      frame "auto" {
        w247 = TRUE  # Save Tunes for Entire Match?
        n137 = Unbundle By Name(w252) -> ("Tune Setpoint"=w249:cluster{"Increment":bool, "Decrement":bool})
        n138 = call "Arm Setpoint FG.vi"("Menu"=fg_typedef."Get") -> ("Setpoint Out"=w248:dbl)  [unwired: 1 in]
        n139 = call "arm tune.vi"("Tune Data"=w249, "Setpoint"=w248, "Save Tunes for Entire Match?"=w247) -> ("Tuned Setpoint"=w246:dbl)  [unwired: 4 in]
      }
      frame "hold position" {
        # "previous auto setpoint (only for code to use, not driver)"
      }
    }
    n140 = feedback-in #4(w101) -> ()
    n141 = disable-structure shown="Enabled" {
      disable-tunnel: w105 -> [w135 w141]
      disable-tunnel: w104 -> [w134 w140]
      disable-tunnel: [w133 w139] -> w103
      frame Disabled {
        # "true = close loop on rate"
        n142 = case shown="True" w135 {
          tunnel: w134 -> [w136 w138]
          tunnel: [w136 w137] -> w133
          frame False {
            # "open loop"
          }
          frame True {
            n143 = call "arm rate pid.vi"("Rate In"=w138) -> ("Rate Out"=w137:dbl)
          }
        }
      }
      frame Enabled {
        n144 = case shown="False" w141 {
          tunnel: w140 -> [w142 w144]
          tunnel: [w142 w143] -> w139
          frame False {
            # "open loop"
          }
          frame True {
            n145 = call "arm pid.vi"("Setpoint"=w144, "Autotune?"=FALSE) -> ("Output"=w143:dbl)
          }
        }
      }
    }
    n146 = feedback #5() -> (w113:T3)
    n147 = feedback-in #5(w113) -> ()
    n148 = case shown="False" w116 {
      tunnel: w115 -> [w147 w151]
      tunnel: w114 -> [w146 w150]
      tunnel: w113 -> [w148 w149]
      frame False {
        n149 = call <vilib>:"WPI_RobotDriveMotors.vi"("RightSpeed"=w146, "LeftSpeed"=w147, "RobotDriveDevRef"=w148) -> ()  [unwired: 6 in, 3 out]
      }
      frame True {
        n150 = call-poly <vilib>:"WPI_RobotDriveArcadeDrive.vi"("Y axis value"=w150, "X axis value"=w151, "RobotDriveDevRef"=w149) -> ()  [unwired: 6 in, 3 out]
      }
    }
    n151 = call "loop timer.vi"() -> ("IPS"=→"Main IPS":dbl, "SPI"=w128:u32)  [unwired: 1 in]
    "Main SPI" <- w128
    n152 = call "performance fg.vi"("Menu"=fg_typedef."Get") -> ("Output"=w125:T24)  [unwired: 1 in]
    n153 = call "combined arm safety.vi"("Input"=w103) -> ("Safe Output"=w102:dbl, "Safety"=w97:cluster{"Arm Safety":bool, "Arm Limit":bool})  [unwired: 13 in]
    n154 = Bundle By Name(cluster=w125, "Main mSPI"=w128) -> (w124:T24)
    n155 = call "Dash Bools.vi"("Input"=w97, "Menu"=fg_typedef."Set") -> ()  [unwired: 1 out]
    n156 = feedback #6() -> (w107:T4)
    n157 = feedback-in #6(w107) -> ()
    n158 = feedback #7() -> (w106:T4)
    n159 = feedback-in #7(w106) -> ()
    n160 = call "performance fg.vi"("Input"=w124, "Menu"=fg_typedef."Set") -> ()  [unwired: 1 out]
    n161 = call <vilib>:"WPI_MotorControlSetOutput.vi"("Output"=w99, "MotorControlDevRef"=w107) -> ()  [unwired: 7 in, 3 out]
    n162 = call <vilib>:"WPI_MotorControlSetOutput.vi"("Output"=w102, "MotorControlDevRef"=w106) -> ()  [unwired: 7 in, 3 out]
  }
  n163 = Merge Errors(w7, "error in", w39, w38, w37, w36, w35, w34, w33, w32, w31, w40, w41) -> (→"error out":errorcluster)
